vi "create_folder.vi"(0 "Name":string, 1 "folder of the day":string="no name", 2 "base path":path, 3 "error in":errorcluster) -> (6 "appended path":path, 9 "error out":errorcluster)   [LabVIEW 2018]
panel:
  out "string":string
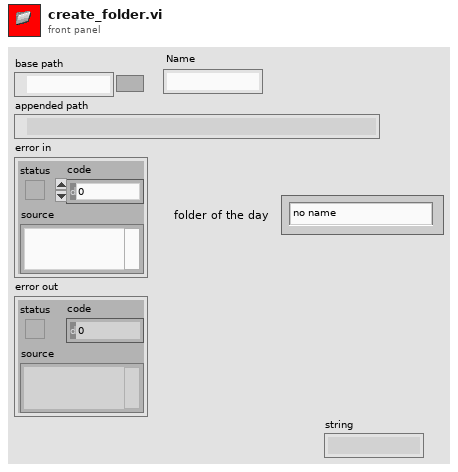
[diagram p1: front panel]
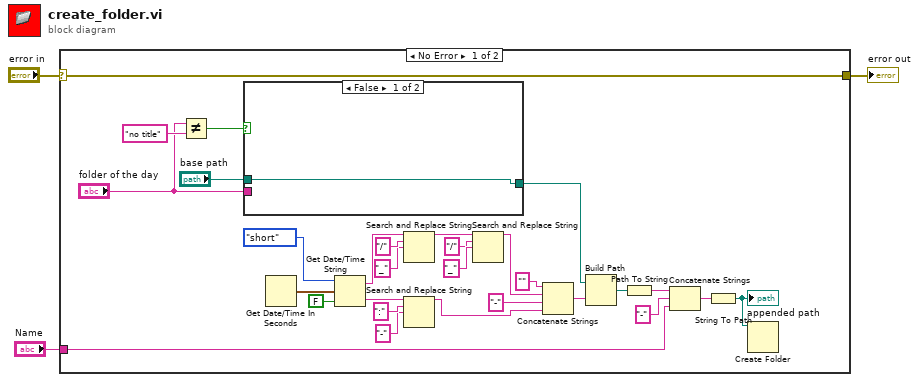
[diagram p0: block diagram]
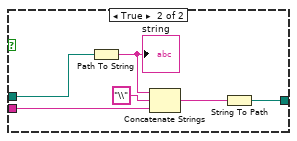
[diagram p2: hidden frame]
diagram:
  n1 = case shown="No Error" "error in" {
    selector: "error in" -> [w32 w40]
    tunnel: [w32 w40] -> w2
    tunnel: "Name" -> [w9 _]
    frame No Error {
      n2 = Not Equal?(x="folder of the day", y="no title") -> (x != y?=w8:bool)
      n3 = case shown="False" w8 {
        tunnel: "base path" -> [w33 w39]
        tunnel: "folder of the day" -> [_ w36]
        tunnel: [w33 w34] -> w4
        frame False {
        }
        frame True {
          n4 = Path To String(path=w39) -> (string=w38:string)
          "string" <- w38
          n5 = Concatenate Strings(w38, "\\" ("string"), w36) -> (w35:string)
          n6 = String To Path(string=w35) -> (path=w34:path)
        }
      }
      n7 = Get Date/Time In Seconds() -> (seconds since 1Jan1904=w30:timestamp)
      n8 = Get Date/Time String(date format (0)=enum16{"short", "long", "abbreviated"}."short", seconds (now)=w30, want seconds? (F)=FALSE) -> (date string=w21:string, time string=w25:string)
      n9 = Search and Replace String(input string=w21, search string="/", replace string="_" ("replace string (\"\")")) -> (result string=w16:string)  [unwired: 5 in, 3 out]
      n10 = Search and Replace String(input string=w25, search string=":", replace string="-" ("replace string (\"\")")) -> (result string=w24:string)  [unwired: 5 in, 3 out]
      n11 = Search and Replace String(input string=w16, search string="/", replace string="_" ("replace string (\"\")")) -> (result string=w15:string)  [unwired: 5 in, 3 out]
      n12 = Concatenate Strings("" ("name or relative path"), w15, "-" ("string"), w24) -> (w29:string)
      n13 = Build Path(base path=w4, name or relative path=w29) -> (appended path=w10:path)
      n14 = Path To String(path=w10) -> (string=w12:string)
      n15 = Concatenate Strings(w12, "-" ("string"), w9) -> (w14:string)
      n16 = String To Path(string=w14) -> (path=w11:path)
      "appended path" <- w11
      n17 = Create Folder(path (use dialog)=w11) -> ()  [unwired: 2 in, 3 out]
    }
    frame Error {
    }
  }
  "error out" <- w2
